vi "Segway - Sobe Rampa.vi"() -> ()   [LabVIEW 2016]
uses:
  <vilib>/NXT/Block Support/NXT_InputPort.ctl
  <vilib>/NXT/Subs/MotorOutput.ctl
  <vilib>/NXT/Block Support/NXT_TimerIndex.ctl
  <vilib>/NXT/Block Support/NXT_OutputPort.ctl
  <vilib>/NXT/Dual Mode Library/Waits/Wait_Num.vi
  <vilib>/NXT/Dual Mode Library/Sensors/EV3_Gyro_Reset.vi
  <vilib>/NXT/Dual Mode Library/Motors/ResetMotor.vi
  <vilib>/NXT/Dual Mode Library/Display/drawNumber.vi
  <vilib>/NXT/Dual Mode Library/Sensors/EV3_Gyro_Rate.vi
  <vilib>/NXT/Dual Mode Library/Motors/Rotation.vi
  <vilib>/NXT/NXTIO Xnodes/NXTIONodeSubVIs/NXTMoveMotors.vi
  <vilib>/NXT/NXTIO Xnodes/AddressXNode/NXTIOAddress.xnode
  <vilib>/NXT/NXTIO Xnodes/NXTIOXNode/NXTIO.xnode
  <vilib>/NXT/Subs/LVHSConnector.ctl
  <vilib>/NXT/LegoClasses/BrickReference/BrickReference.lvclass
panel:
  in  "stop":bool
  out "e":dbl
  out "Waveform Chart 2":dbl(graph)
  out "b":dbl
  out "a":dbl
  in  "dt_program_flow":dbl
  out "dt":dbl
  out "timer_time":dbl
  out "EncSum":dbl
  out "VelAngRoda2":dbl(graph)
  out "PosAngRoda2":dbl(graph)
  out "PosAngCorpo2":dbl(graph)
  out "VelAngCorpo2":dbl(graph)
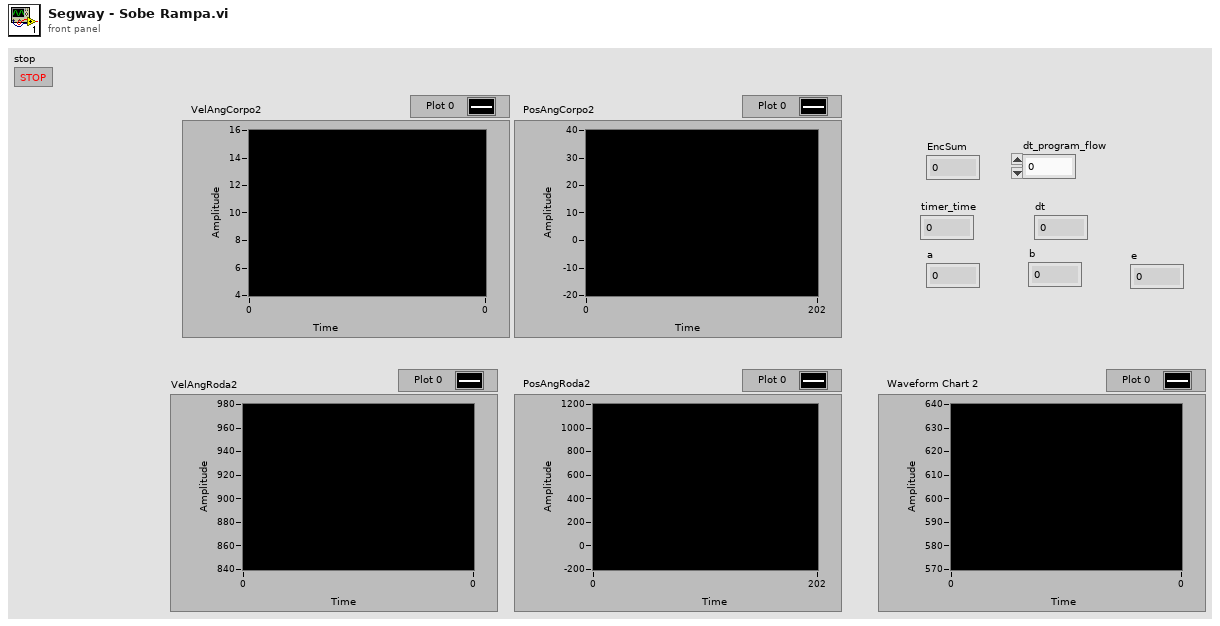
[diagram p1: front panel]
types:
  T1 = typedef "NXT_TimerIndex.ctl" = u8
  T2 = typedef "MotorOutput.ctl" = u8
  T3 = typedef "NXT_InputPort.ctl" = u32
  T4 = typedef "LVHSConnector.ctl" = refnum<class "BrickReference.lvclass">
  T5 = typedef "NXT_OutputPort.ctl" = u8
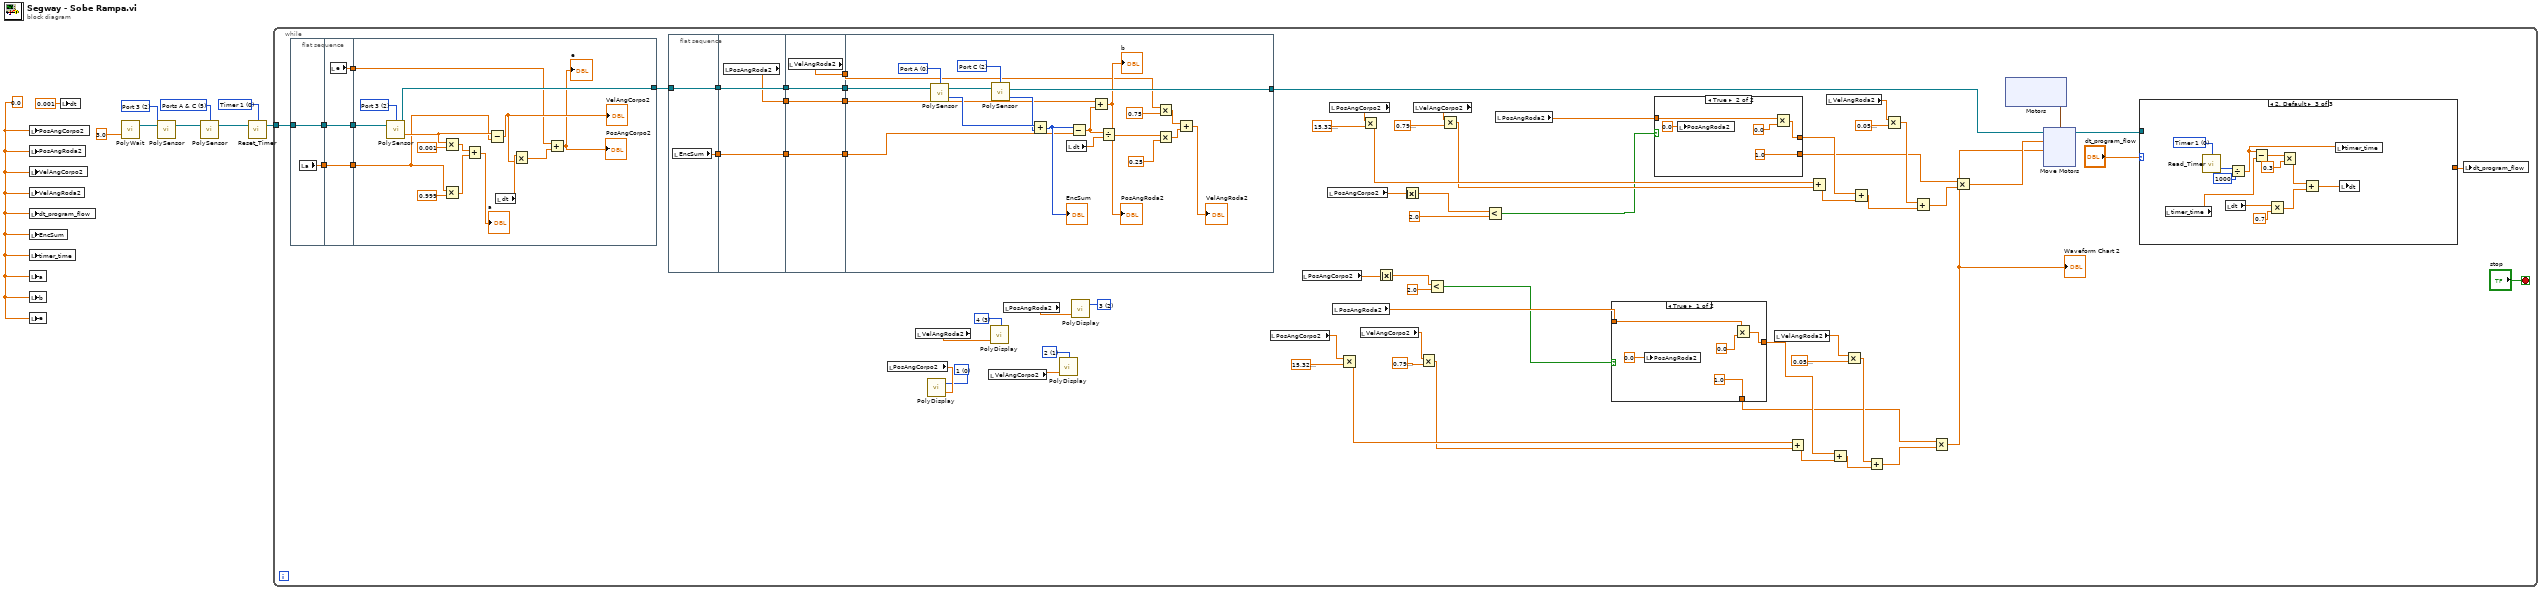
[diagram p0: block diagram]
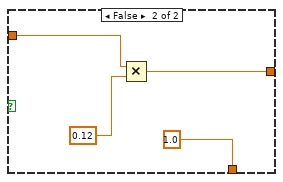
[diagram p2: hidden frame]
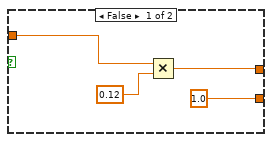
[diagram p3: hidden frame]
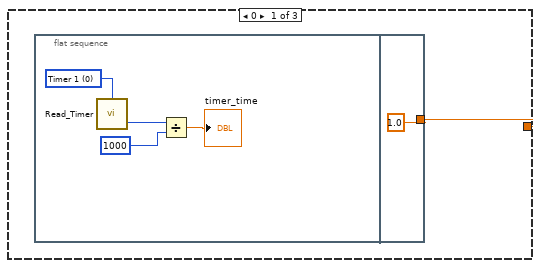
[diagram p4: hidden frame]
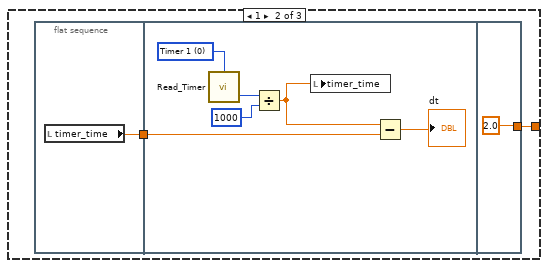
[diagram p5: hidden frame]
diagram:
  w3 = T1 0 items=["Timer 1", "Timer 2", "Timer 3"] ("Timer (Timer 1)")
  w8 = T2 5 items=["Port A"=0, "Port B"=1, "Port C"=2, "Ports A & B"=4, "Ports A & C"=5, "Ports B & C"=6, "All Ports"=3] ("Port (All Ports)")
  w9 = T3 2 items=["Port 1", "Port 2", "Port 3", "Port 4"] ("Port (Port 1)")
  w5 = 0.0 ("PosAngCorpo2")
  n1 = local write "PosAngCorpo2"(w5) -> ()
  n2 = local write "PosAngRoda2"(w5) -> ()
  n3 = local write "VelAngCorpo2"(w5) -> ()
  n4 = local write "VelAngRoda2"(w5) -> ()
  n5 = local write "dt_program_flow"(w5) -> ()
  n6 = local write "EncSum"(w5) -> ()
  n7 = local write "timer_time"(w5) -> ()
  n8 = local write "a"(w5) -> ()
  n9 = local write "b"(w5) -> ()
  n10 = local write "e"(w5) -> ()
  n11 = local write "dt"(0.001 ("dt")) -> ()
  n12 = call-poly <vilib>:"PolyWait.vi"("Time (1 sec)"=sgl 3.0) -> ("NXT/EV3"=w4:T4)  [unwired: 3 in]
  n13 = call-poly <vilib>:"PolySensor.vi"("NXT/EV3"=w4, "Port (Port 1)"=w9) -> ("NXT/EV3"=w7:T4)  [unwired: 2 in]
  n14 = call-poly <vilib>:"PolySensor.vi"("NXT/EV3"=w7, "Port (All Ports)"=w8) -> ("NXT/EV3"=w1:T4)  [unwired: 2 in]
  n15 = call <vilib>:"Reset_Timer.vi"("NXT/EV3"=w1, "Timer (Timer 1)"=w3) -> ("NXT/EV3"=w2:T4)  [unwired: 2 in]
  n16 = while {
    tunnel: w2 -> [w68]
    stop <- "stop" stop-if-true
    w43 = i16 2 items=["1", "2", "3", "4", "5", "6", "7", "8", "9", "10", "11", "12"] ("Line")
    w44 = i16 3 items=["1", "2", "3", "4", "5", "6", "7", "8", "9", "10", "11", "12"] ("Line")
    w45 = i16 1 items=["1", "2", "3", "4", "5", "6", "7", "8", "9", "10", "11", "12"] ("Line")
    w47 = i16 0 items=["1", "2", "3", "4", "5", "6", "7", "8", "9", "10", "11", "12"] ("Line")
    n17 = flat-sequence {
      tunnel: w68 -> [w129]
      tunnel: [w129] -> w62
      tunnel: [w128] -> w60
      tunnel: w62 -> [w132]
      tunnel: [w132] -> w61
      tunnel: w60 -> [w131]
      tunnel: [w131] -> w59
      tunnel: [w130] -> w58
      tunnel: [w139] -> w71
      tunnel: w61 -> [w135]
      tunnel: w59 -> [w134]
      tunnel: w58 -> [w133]
      frame #0 {
        n18 = local read "a"() -> (w128:dbl)
      }
      frame #1 {
        n19 = local read "e"() -> (w130:dbl)
      }
      frame #2 {
        w143 = T3 2 items=["Port 1", "Port 2", "Port 3", "Port 4"] ("Port (Port 1)")
        n20 = call-poly <vilib>:"PolySensor.vi"("NXT/EV3"=w135, "Port (Port 1)"=w143) -> ("Degrees/Second"=w142:sgl, "NXT/EV3"=w139:T4)  [unwired: 1 in]
        n21 = Multiply(x=w142, y=0.001) -> (x*y=w145:dbl)
        n22 = Multiply(x=w134, y=0.999) -> (x*y=w138:dbl)
        n23 = Add(x=w145, y=w138) -> (x+y=→"a":dbl)
        n24 = Subtract(x=w142, y=w134) -> (x-y=w140:dbl)
        "VelAngCorpo2" <- w140
        n25 = local read "dt"() -> (w141:dbl)
        n26 = Multiply(x=w141, y=w140) -> (x*y=w144:dbl)
        n27 = Add(x=w133, y=w144) -> (x+y=→"PosAngCorpo2" →"e":dbl)
      }
    }
    n28 = flat-sequence {
      tunnel: w71 -> [w100]
      tunnel: [w100] -> w57
      tunnel: [w99] -> w56
      tunnel: w57 -> [w103]
      tunnel: [w103] -> w55
      tunnel: w56 -> [w102]
      tunnel: [w102] -> w53
      tunnel: [w101] -> w50
      tunnel: w55 -> [w107]
      tunnel: [w107] -> w54
      tunnel: w53 -> [w106]
      tunnel: [w106] -> w52
      tunnel: [w105] -> w51
      tunnel: w50 -> [w104]
      tunnel: [w104] -> w49
      tunnel: w54 -> [w116]
      tunnel: [w114] -> w70
      tunnel: w52 -> [w110]
      tunnel: w51 -> [w109]
      tunnel: w49 -> [w108]
      frame #0 {
        n29 = local read "EncSum"() -> (w99:dbl)
      }
      frame #1 {
        n30 = local read "PosAngRoda2"() -> (w101:dbl)
      }
      frame #2 {
        n31 = local read "VelAngRoda2"() -> (w105:dbl)
      }
      frame #3 {
        w118 = T5 2 items=["Port A", "Port B", "Port C", "Port D"] ("Port (Port A)")
        w121 = T5 0 items=["Port A", "Port B", "Port C", "Port D"] ("Port (Port A)")
        n32 = call-poly <vilib>:"PolySensor.vi"("NXT/EV3"=w116, "Port (Port A)"=w121) -> ("Angle of Rotation"=w120:i32, "NXT/EV3"=w115:T4)  [unwired: 1 in]
        n33 = call-poly <vilib>:"PolySensor.vi"("NXT/EV3"=w115, "Port (Port A)"=w118) -> ("Angle of Rotation"=w117:i32, "NXT/EV3"=w114:T4)  [unwired: 1 in]
        n34 = Add(x=w120, y=w117) -> (x+y=w127:i32)
        "EncSum" <- w127
        n35 = local read "dt"() -> (w119:dbl)
        n36 = Subtract(x=w127, y=w110) -> (x-y=w126:dbl)
        n37 = Add(x=w108, y=w126) -> (x+y=→"PosAngRoda2" →"b":dbl)
        n38 = Divide(x=w126, y=w119) -> (x/y=w122:dbl)
        n39 = Multiply(x=w109, y=0.75) -> (x*y=w112:dbl)
        n40 = Multiply(x=w122, y=sgl 0.25) -> (x*y=w124:dbl)
        n41 = Add(x=w112, y=w124) -> (x+y=→"VelAngRoda2":dbl)
      }
    }
    n42 = local read "PosAngCorpo2"() -> (w48:dbl)
    n43 = local read "VelAngRoda2"() -> (w41:dbl)
    n44 = call-poly <vilib>:"PolyDisplay.vi"("number"=w48, "Line"=w47) -> ()  [unwired: 2 in, 1 out]
    n45 = local read "VelAngCorpo2"() -> (w46:dbl)
    n46 = call-poly <vilib>:"PolyDisplay.vi"("number"=w41, "Line"=w44) -> ()  [unwired: 2 in, 1 out]
    n47 = local read "PosAngRoda2"() -> (w42:dbl)
    n48 = call-poly <vilib>:"PolyDisplay.vi"("number"=w46, "Line"=w45) -> ()  [unwired: 2 in, 1 out]
    n49 = call-poly <vilib>:"PolyDisplay.vi"("number"=w42, "Line"=w43) -> ()  [unwired: 2 in, 1 out]
    n50 = local read "PosAngCorpo2"() -> (w25:dbl)
    n51 = local read "PosAngCorpo2"() -> (w17:dbl)
    n52 = local read "PosAngCorpo2"() -> (w20:dbl)
    n53 = local read "PosAngCorpo2"() -> (w74:dbl)
    n54 = local read "PosAngRoda2"() -> (w23:dbl)
    n55 = Multiply(x=w25, y=sgl 15.33) -> (x*y=w32:dbl)
    n56 = local read "VelAngCorpo2"() -> (w26:dbl)
    n57 = Multiply(x=w74, y=sgl 15.33) -> (x*y=w67:dbl)
    n58 = Absolute Value(x=w17) -> (abs(x)=w16:dbl)
    n59 = Absolute Value(x=w20) -> (abs(x)=w19:dbl)
    n60 = local read "VelAngCorpo2"() -> (w73:dbl)
    n61 = Multiply(x=w26, y=sgl 0.79) -> (x*y=w31:dbl)
    n62 = Less?(x=w16, y=2.0) -> (x < y?=w14:bool)
    n63 = Multiply(x=w73, y=sgl 0.79) -> (x*y=w66:dbl)
    n64 = Less?(x=w19, y=2.0) -> (x < y?=w13:bool)
    n65 = local read "PosAngRoda2"() -> (w39:dbl)
    n66 = case shown="True" w14 {
      tunnel: w23 -> [w83 w88]
      tunnel: [w82 w87] -> w22
      tunnel: [1.0 1.0 ("y")] -> w21
      frame True {
        n67 = local write "PosAngRoda2"(0.0) -> ()
        n68 = Multiply(x=w83, y=0.0) -> (x*y=w82:dbl)
      }
      frame False {
        n69 = Multiply(x=w88, y=0.12) -> (x*y=w87:dbl)
      }
    }
    n70 = case shown="True" w13 {
      tunnel: w39 -> [w93 w97]
      tunnel: [w91 w96] -> w38
      tunnel: [1.0 ("y") 1.0 ("y")] -> w37
      frame False {
        n71 = Multiply(x=w93, y=0.12) -> (x*y=w91:dbl)
      }
      frame True {
        n72 = local write "PosAngRoda2"(0.0 ("PosAngRoda2")) -> ()
        n73 = Multiply(x=w97, y=0.0) -> (x*y=w96:dbl)
      }
    }
    n74 = local read "VelAngRoda2"() -> (w24:dbl)
    n75 = Add(x=w32, y=w31) -> (x+y=w30:dbl)
    n76 = Add(x=w67, y=w66) -> (x+y=w65:dbl)
    n77 = local read "VelAngRoda2"() -> (w72:dbl)
    n78 = Add(x=w22, y=w30) -> (x+y=w29:dbl)
    n79 = Multiply(x=w24, y=sgl 0.06) -> (x*y=w28:dbl)
    n80 = Add(x=w38, y=w65) -> (x+y=w64:dbl)
    n81 = Add(x=w28, y=w29) -> (x+y=w27:dbl)
    n82 = Multiply(x=w72, y=sgl 0.06) -> (x*y=w63:dbl)
    n83 = Add(x=w63, y=w64) -> (x+y=w36:dbl)
    n84 = Multiply(x=w21, y=w27) -> (x*y=w11:dbl)
    "Waveform Chart 2" <- w11
    n85 = Multiply(x=w37, y=w36) -> (x*y=w12:dbl)
    n86 = xnode "Motors"() -> ("Motor"=w78:cluster{"Port":T5, "Port":T5})
    n87 = xnode "Move Motors"("Power/Speed 2"=w11, "Power/Speed 1"=w12, "Motors"=w78, "NXT/EV3"=w70) -> ("NXT/EV3"=w69:T4)
    n88 = case shown="2, Default" "dt_program_flow" {
      tunnel: [w157 w163 _] -> w80
      tunnel: w69 -> [_ _ _]
      frame 0 {
        n89 = flat-sequence {
          tunnel: [1.0 ("dt_program_flow")] -> w157
          frame #0 {
            w161 = T1 0 items=["Timer 1", "Timer 2", "Timer 3"] ("Timer (Timer 1)")
            n90 = call <vilib>:"Read_Timer.vi"("Timer (Timer 1)"=w161) -> ("Value (msec)"=w158:u32)  [unwired: 2 in, 1 out]
            n91 = Divide(x=w158, y=u32 1000) -> (x/y=→"timer_time":dbl)
          }
          frame #1 {
          }
        }
      }
      frame 1 {
        n92 = flat-sequence {
          tunnel: [w165] -> w164
          tunnel: w164 -> [w171]
          tunnel: [2.0 ("dt_program_flow")] -> w163
          frame #0 {
            n93 = local read "timer_time"() -> (w165:dbl)
          }
          frame #1 {
            w169 = T1 0 items=["Timer 1", "Timer 2", "Timer 3"] ("Timer (Timer 1)")
            n94 = call <vilib>:"Read_Timer.vi"("Timer (Timer 1)"=w169) -> ("Value (msec)"=w168:u32)  [unwired: 2 in, 1 out]
            n95 = Divide(x=w168, y=u32 1000) -> (x/y=w166:dbl)
            n96 = local write "timer_time"(w166) -> ()
            n97 = Subtract(x=w166, y=w171) -> (x-y=→"dt":dbl)
          }
          frame #2 {
          }
        }
      }
      frame 2, Default {
        w176 = T1 0 items=["Timer 1", "Timer 2", "Timer 3"] ("Timer (Timer 1)")
        n98 = local read "timer_time"() -> (w173:dbl)
        n99 = call <vilib>:"Read_Timer.vi"("Timer (Timer 1)"=w176) -> ("Value (msec)"=w175:u32)  [unwired: 2 in, 1 out]
        n100 = local read "dt"() -> (w178:dbl)
        n101 = Divide(x=w175, y=u32 1000) -> (x/y=w183:dbl)
        n102 = Subtract(x=w183, y=w173) -> (x-y=w182:dbl)
        n103 = Multiply(x=w178, y=0.7) -> (x*y=w177:dbl)
        n104 = Multiply(x=w182, y=0.3) -> (x*y=w180:dbl)
        n105 = Add(x=w180, y=w177) -> (x+y=w184:dbl)
        n106 = local write "timer_time"(w183) -> ()
        n107 = local write "dt"(w184) -> ()
      }
    }
    n108 = local write "dt_program_flow"(w80) -> ()
  }
